vi "InitializeAOTFOutput.vi"(0 "% puls-duration":dbl=95.0, 1 "Timing Info":T2 {"#s" format="%.2e"; "Fs" format="%.2e"}, 2 "AOTF":u16(ring) items=["None", "Laser 1", "Laser 2", "Laser 1 + 2", "Laser 3", "Laser 1 + 3", "Laser 2 + 3", "Laser 1+2+3", "Laser 1+2+3+4", "Laser 2+3+4"], 3 "Image Settings":T3={"Start Position (µm)"={"x"=0.0, "y"=0.0, "z"=0.0}, "End Position (µm)"={"x"=10.0, "y"=10.0, "z"=0.0}, "Image Resolution (nm/pixel)"={"x"=50.0, "y"=50.0, "z"=100.0}, "Image Size (µm)"={"x"=10.0, "y"=10.0, "z"=0.0}, "Image Size (pixel)"={"x"=50, "y"=50, "z"=0}, "Time Resolution\n(ms/pixel)"=7.0, "1st Axis"=0, "2nd Axis"=1, "Retrace"=FALSE, "Estimated Time"=""} {"2nd Axis" items=["x", "y", "z"]; "1st Axis" items=["x", "y", "z"]; "Time Resolution\n(ms/pixel)" format="%.2f"; "Image Resolution (nm/pixel)"."z" format="%.2f"; "Image Resolution (nm/pixel)"."y" format="%.2f"; "Image Resolution (nm/pixel)"."x" format="%.2f"; "Image Size (µm)"."z" format="%.2f"; "Image Size (µm)"."y" format="%.2f"; "Image Size (µm)"."x" format="%.2f"; "End Position (µm)"."z" format="%.2f"; "End Position (µm)"."y" format="%.2f"; "End Position (µm)"."x" format="%.2f"; "Start Position (µm)"."z" format="%.2f"; "Start Position (µm)"."y" format="%.2f"; "Start Position (µm)"."x" format="%.2f"}, 4 "% rel. duration":u8=50 min=1 max=99) -> (5 "Array":T1[](array[typedef]))   [LabVIEW 2009]
uses:
  ImageSettings.ctt
  TimingInfo.ctt
  AnalogTrace.ctt
panel:
  in  "Trace":T1
  out "Frequency":dbl format="%.2e"
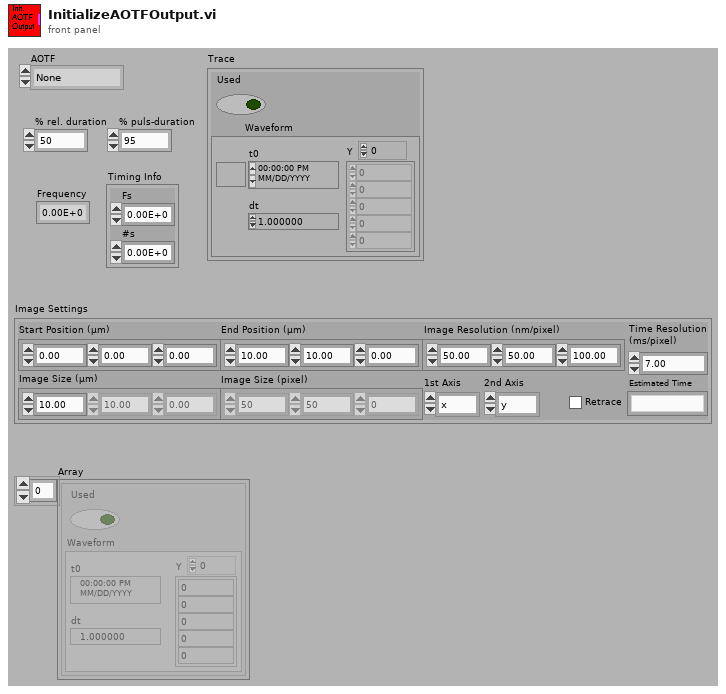
[diagram p1: front panel]
types:
  T1 = typedef "AnalogTrace.ctt" = cluster{"Used":bool, "Waveform":waveform(dbl)}
  T2 = typedef "TimingInfo.ctt" = cluster{"Fs":dbl, "#s":dbl}
  T3 = typedef "ImageSettings.ctt" = cluster{"Start Position (µm)":cluster{"x":dbl, "y":dbl, "z":dbl}, "End Position (µm)":cluster{"x":dbl, "y":dbl, "z":dbl}, "Image Resolution (nm/pixel)":cluster{"x":dbl, "y":dbl, "z":dbl}, "Image Size (µm)":cluster{"x":dbl, "y":dbl, "z":dbl}, "Image Size (pixel)":cluster{"x":u32, "y":u32, "z":u32}, "Time Resolution\n(ms/pixel)":dbl, "1st Axis":u16, "2nd Axis":u16, "Retrace":bool, "Estimated Time":string}
  T4 = typedef "AOTFSettings.ctt" = cluster{"Laser 1 Output Channel":tag, "AOTF  1 Output Voltage":dbl, "Laser 2 Output Channel":tag, "AOTF  2 Output Voltage":dbl, "Laser 3 Output Channel":tag, "AOTF  3 Output Voltage":dbl, "Pixel per Cycle":u16, "Time per Cycle  / ms":dbl, "Laser 4 Output Channel":tag, "AOTF  4 Output Voltage":dbl}
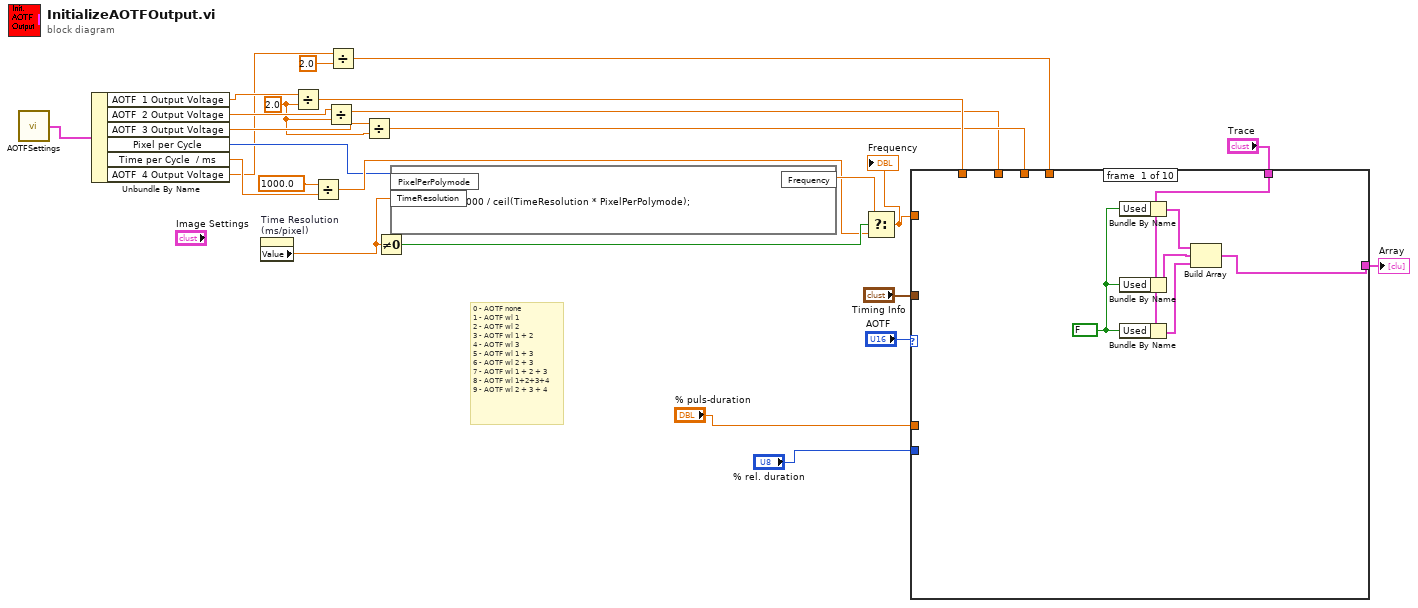
[diagram p0: block diagram]
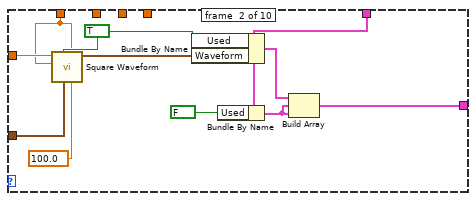
[diagram p2: hidden frame]
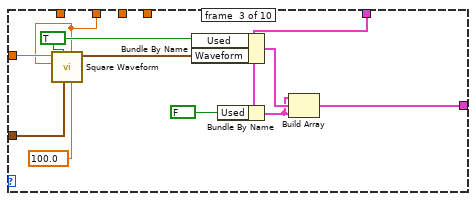
[diagram p3: hidden frame]
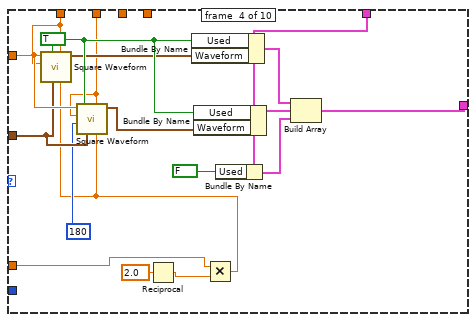
[diagram p4: hidden frame]
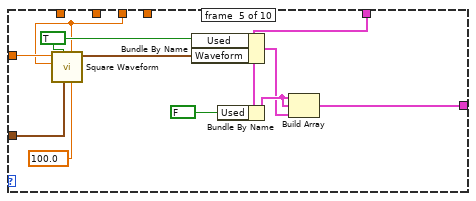
[diagram p5: hidden frame]
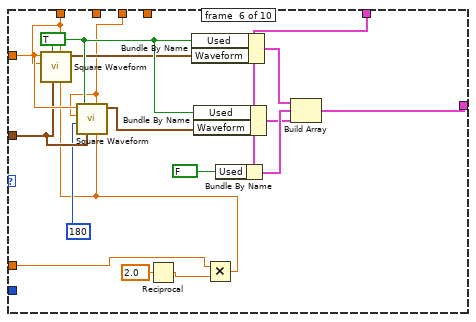
[diagram p6: hidden frame]
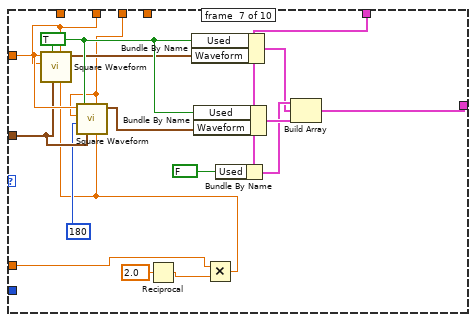
[diagram p7: hidden frame]
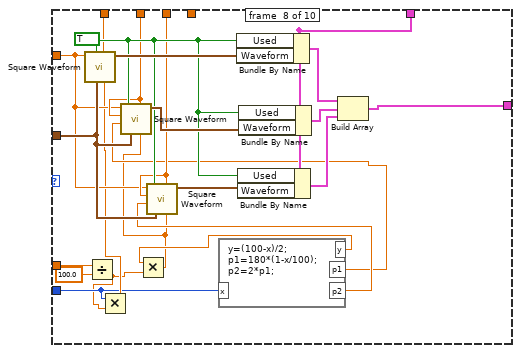
[diagram p8: hidden frame]
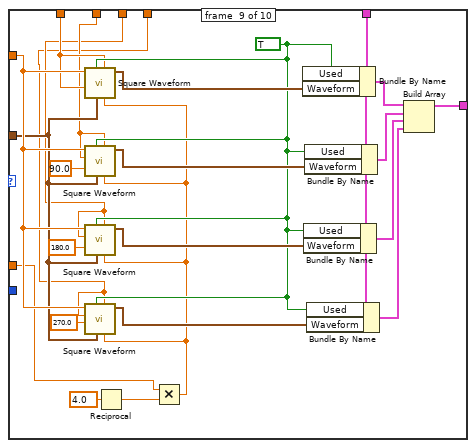
[diagram p9: hidden frame]
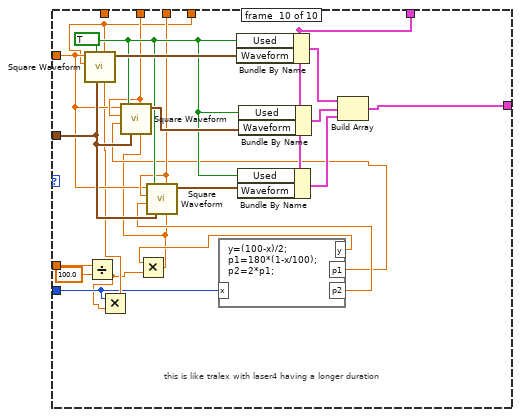
[diagram p10: hidden frame]
diagram:
  w8 = 2.0 ("y")
  # "0 - AOTF none\n1 - AOTF wl 1\n2 - AOTF wl 2\n3 - AOTF wl 1 + 2\n4 - AOTF wl 3\n5 - AOTF wl 1 + 3\n6 - AOTF wl 2 + 3\n7 - AOTF wl 1 + 2 + 3\n8 - AOTF wl 1+2+3+4\n9 - AOTF wl 2 + 3 + 4"
  n1 = call "AOTFSettings.vi"() -> ("AOTF Setting (Output)"=w16:T4)  [unwired: 2 in]
  n2 = Unbundle By Name(w16) -> ("AOTF  1 Output Voltage"=w15:dbl, "AOTF  2 Output Voltage"=w10:dbl, "AOTF  3 Output Voltage"=w12:dbl, "Pixel per Cycle"=w14:u16, "Time per Cycle  / ms"=w7:dbl, "AOTF  4 Output Voltage"=w2:dbl)
  n3 = property on="Time Resolution\n(ms/pixel)" class="Digital (strict)"() -> ("Value"=w23:dbl)  [unwired: 2 in, 2 out]
  n4 = Divide(x=w15, y=w8) -> (x/y=w13:dbl)
  n5 = Divide(x=1000.0 ("y"), y=w7) -> (x/y=w19:dbl)
  n6 = Divide(x=w10, y=w8) -> (x/y=w9:dbl)
  n7 = Divide(x=w2, y=2.0) -> (x/y=w1:dbl)
  n8 = Divide(x=w12, y=w8) -> (x/y=w11:dbl)
  n9 = Not Equal To 0?(x=w23) -> (x != 0?=w24:bool)
  n10 = formula code="Frequency =1000 / ceil(TimeResolution * PixelPerPolymode);"("PixelPerPolymode"=w14, "TimeResolution"=w23) -> ("Frequency"=w22:dbl)
  n11 = Select(t=w22, s=w24, f=w19) -> (s? t:f=w21:dbl)
  "Frequency" <- w21
  n12 = case shown="9" "AOTF" {
    tunnel: w21 -> [_ w42 w53 w71 w82 w100 w118 w130 w159 w178]
    tunnel: "Timing Info" -> [_ w41 w52 w70 w81 w99 w117 w139 w153 w186]
    tunnel: "Trace" -> [w31 w35 w47 w67 w76 w96 w114 w140 w161 w187]
    tunnel: w13 -> [_ w34 _ w62 _ w91 _ w133 w148 _]
    tunnel: [w29 w36 w48 w64 w77 w93 w112 w135 w162 w182] -> w17
    tunnel: w9 -> [_ _ w43 w61 _ _ w101 w132 w147 w180]
    tunnel: w11 -> [_ _ _ _ w72 w83 w102 w131 w146 w179]
    tunnel: "% rel. duration" -> [_ _ _ _ _ _ _ w122 _ w170]
    tunnel: "% puls-duration" -> [_ _ _ w55 _ w87 w107 w124 w150 w172]
    tunnel: w1 -> [_ _ _ _ _ _ _ _ w145 w166]
    frame #0 {
      w26 = FALSE ("Used")
      n13 = Bundle By Name(cluster=w31, "Used"=w26) -> (w30:T1)
      n14 = Bundle By Name(cluster=w31, "Used"=w26) -> (w28:T1)
      n15 = Bundle By Name(cluster=w31, "Used"=w26) -> (w27:T1)
      n16 = Build Array(w30, w28, w27) -> (w29:T1[])
    }
    frame #1 {
      w40 = TRUE ("reset signal")
      n17 = call "Square Waveform.vi"("duty cycle (%)"=100.0, "offset"=w34, "sampling info"=w41, "reset signal"=w40, "amplitude"=w34, "frequency"=w42) -> ("signal out"=w33:waveform(dbl))  [unwired: 4 in, 1 out]
      n18 = Bundle By Name(cluster=w35, "Used"=w40, "Waveform"=w33) -> (w37:T1)
      n19 = Bundle By Name(cluster=w35, "Used"=FALSE) -> (w32:T1)
      n20 = Build Array(w37, w32, w32) -> (w36:T1[])
    }
    frame #2 {
      w51 = TRUE ("reset signal")
      n21 = call "Square Waveform.vi"("duty cycle (%)"=100.0, "offset"=w43, "sampling info"=w52, "reset signal"=w51, "amplitude"=w43, "frequency"=w53) -> ("signal out"=w46:waveform(dbl))  [unwired: 4 in, 1 out]
      n22 = Bundle By Name(cluster=w47, "Used"=w51, "Waveform"=w46) -> (w45:T1)
      n23 = Bundle By Name(cluster=w47, "Used"=FALSE) -> (w44:T1)
      n24 = Build Array(w44, w45, w44) -> (w48:T1[])
    }
    frame #3 {
      w69 = TRUE ("reset signal")
      n25 = Reciprocal(x=2.0) -> (1/x=w57:dbl)
      n26 = Multiply(x=w55, y=w57) -> (x*y=w54:dbl)
      n27 = call "Square Waveform.vi"("duty cycle (%)"=w54, "offset"=w62, "sampling info"=w70, "reset signal"=w69, "amplitude"=w62, "frequency"=w71) -> ("signal out"=w68:waveform(dbl))  [unwired: 4 in, 1 out]
      n28 = call "Square Waveform.vi"("duty cycle (%)"=w54, "offset"=w61, "sampling info"=w70, "reset signal"=w69, "phase"=u8 180, "amplitude"=w61, "frequency"=w71) -> ("signal out"=w63:waveform(dbl))  [unwired: 3 in, 1 out]
      n29 = Bundle By Name(cluster=w67, "Used"=w69, "Waveform"=w68) -> (w65:T1)
      n30 = Bundle By Name(cluster=w67, "Used"=w69, "Waveform"=w63) -> (w60:T1)
      n31 = Bundle By Name(cluster=w67, "Used"=FALSE) -> (w59:T1)
      n32 = Build Array(w65, w60, w59) -> (w64:T1[])
    }
    frame #4 {
      w80 = TRUE ("reset signal")
      n33 = call "Square Waveform.vi"("duty cycle (%)"=100.0, "offset"=w72, "sampling info"=w81, "reset signal"=w80, "amplitude"=w72, "frequency"=w82) -> ("signal out"=w75:waveform(dbl))  [unwired: 4 in, 1 out]
      n34 = Bundle By Name(cluster=w76, "Used"=w80, "Waveform"=w75) -> (w73:T1)
      n35 = Bundle By Name(cluster=w76, "Used"=FALSE) -> (w74:T1)
      n36 = Build Array(w74, w74, w73) -> (w77:T1[])
    }
    frame #5 {
      w98 = TRUE ("reset signal")
      n37 = Reciprocal(x=2.0) -> (1/x=w89:dbl)
      n38 = Multiply(x=w87, y=w89) -> (x*y=w86:dbl)
      n39 = call "Square Waveform.vi"("duty cycle (%)"=w86, "offset"=w91, "sampling info"=w99, "reset signal"=w98, "amplitude"=w91, "frequency"=w100) -> ("signal out"=w97:waveform(dbl))  [unwired: 4 in, 1 out]
      n40 = call "Square Waveform.vi"("duty cycle (%)"=w86, "offset"=w83, "sampling info"=w99, "reset signal"=w98, "phase"=u8 180, "amplitude"=w83, "frequency"=w100) -> ("signal out"=w92:waveform(dbl))  [unwired: 3 in, 1 out]
      n41 = Bundle By Name(cluster=w96, "Used"=w98, "Waveform"=w97) -> (w94:T1)
      n42 = Bundle By Name(cluster=w96, "Used"=w98, "Waveform"=w92) -> (w84:T1)
      n43 = Bundle By Name(cluster=w96, "Used"=FALSE) -> (w85:T1)
      n44 = Build Array(w94, w85, w84) -> (w93:T1[])
    }
    frame #6 {
      w116 = TRUE ("reset signal")
      n45 = Reciprocal(x=2.0) -> (1/x=w109:dbl)
      n46 = Multiply(x=w107, y=w109) -> (x*y=w106:dbl)
      n47 = call "Square Waveform.vi"("duty cycle (%)"=w106, "offset"=w101, "sampling info"=w117, "reset signal"=w116, "amplitude"=w101, "frequency"=w118) -> ("signal out"=w115:waveform(dbl))  [unwired: 4 in, 1 out]
      n48 = call "Square Waveform.vi"("duty cycle (%)"=w106, "offset"=w102, "sampling info"=w117, "reset signal"=w116, "phase"=u8 180, "amplitude"=w102, "frequency"=w118) -> ("signal out"=w111:waveform(dbl))  [unwired: 3 in, 1 out]
      n49 = Bundle By Name(cluster=w114, "Used"=w116, "Waveform"=w115) -> (w103:T1)
      n50 = Bundle By Name(cluster=w114, "Used"=w116, "Waveform"=w111) -> (w105:T1)
      n51 = Bundle By Name(cluster=w114, "Used"=FALSE) -> (w104:T1)
      n52 = Build Array(w104, w103, w105) -> (w112:T1[])
    }
    frame #7 {
      w137 = TRUE ("reset signal")
      n53 = Divide(x=w124, y=100.0) -> (x/y=w121:dbl)
      n54 = Multiply(x=w122, y=w121) -> (x*y=w125:dbl)
      n55 = call "Square Waveform.vi"("duty cycle (%)"=w125, "offset"=w133, "sampling info"=w139, "reset signal"=w137, "amplitude"=w133, "frequency"=w130) -> ("signal out"=w141:waveform(dbl))  [unwired: 4 in, 1 out]
      n56 = formula code="y=(100-x)/2;\np1=180*(1-x/100);\np2=2*p1;"("x"=w122) -> ("y"=w120:dbl, "p1"=w126:dbl, "p2"=w127:dbl)
      n57 = Multiply(x=w120, y=w121) -> (x*y=w119:dbl)
      n58 = call "Square Waveform.vi"("duty cycle (%)"=w119, "offset"=w132, "sampling info"=w139, "reset signal"=w137, "phase"=w126, "amplitude"=w132, "frequency"=w130) -> ("signal out"=w138:waveform(dbl))  [unwired: 3 in, 1 out]
      n59 = call "Square Waveform.vi"("duty cycle (%)"=w119, "offset"=w131, "sampling info"=w139, "reset signal"=w137, "phase"=w127, "amplitude"=w131, "frequency"=w130) -> ("signal out"=w134:waveform(dbl))  [unwired: 3 in, 1 out]
      n60 = Bundle By Name(cluster=w140, "Used"=w137, "Waveform"=w141) -> (w136:T1)
      n61 = Bundle By Name(cluster=w140, "Used"=w137, "Waveform"=w134) -> (w129:T1)
      n62 = Bundle By Name(cluster=w140, "Used"=w137, "Waveform"=w138) -> (w128:T1)
      n63 = Build Array(w136, w128, w129) -> (w135:T1[])
    }
    frame #8 {
      w154 = TRUE
      n64 = Reciprocal(x=4.0) -> (1/x=w152:dbl)
      n65 = Multiply(x=w150, y=w152) -> (x*y=w149:dbl)
      n66 = call "Square Waveform.vi"("duty cycle (%)"=w149, "offset"=w148, "sampling info"=w153, "reset signal"=w154, "phase"=w148, "frequency"=w159) -> ("signal out"=w158:waveform(dbl))  [unwired: 4 in, 1 out]
      n67 = call "Square Waveform.vi"("duty cycle (%)"=w149, "offset"=w147, "sampling info"=w153, "reset signal"=w154, "phase"=90.0 ("amplitude"), "amplitude"=w147, "frequency"=w159) -> ("signal out"=w157:waveform(dbl))  [unwired: 3 in, 1 out]
      n68 = call "Square Waveform.vi"("duty cycle (%)"=w149, "offset"=w146, "sampling info"=w153, "reset signal"=w154, "phase"=180.0 ("amplitude"), "amplitude"=w146, "frequency"=w159) -> ("signal out"=w156:waveform(dbl))  [unwired: 3 in, 1 out]
      n69 = call "Square Waveform.vi"("duty cycle (%)"=w149, "offset"=w145, "sampling info"=w153, "reset signal"=w154, "phase"=270.0 ("amplitude"), "amplitude"=w145, "frequency"=w159) -> ("signal out"=w155:waveform(dbl))  [unwired: 3 in, 1 out]
      n70 = Bundle By Name(cluster=w161, "Used"=w154, "Waveform"=w158) -> (w163:T1)
      n71 = Bundle By Name(cluster=w161, "Used"=w154, "Waveform"=w156) -> (w164:T1)
      n72 = Bundle By Name(cluster=w161, "Used"=w154, "Waveform"=w157) -> (w165:T1)
      n73 = Bundle By Name(cluster=w161, "Used"=w154, "Waveform"=w155) -> (w160:T1)
      n74 = Build Array(w163, w165, w164, w160) -> (w162:T1[])
    }
    frame #9 {
      w184 = TRUE ("reset signal")
      # "this is like tralex with laser4 having a longer duration"
      n75 = Divide(x=w172, y=100.0) -> (x/y=w169:dbl)
      n76 = Multiply(x=w170, y=w169) -> (x*y=w173:dbl)
      n77 = call "Square Waveform.vi"("duty cycle (%)"=w173, "offset"=w166, "sampling info"=w186, "reset signal"=w184, "amplitude"=w166, "frequency"=w178) -> ("signal out"=w188:waveform(dbl))  [unwired: 4 in, 1 out]
      n78 = formula code="y=(100-x)/2;\np1=180*(1-x/100);\np2=2*p1;"("x"=w170) -> ("y"=w168:dbl, "p1"=w174:dbl, "p2"=w175:dbl)
      n79 = Multiply(x=w168, y=w169) -> (x*y=w167:dbl)
      n80 = call "Square Waveform.vi"("duty cycle (%)"=w167, "offset"=w180, "sampling info"=w186, "reset signal"=w184, "phase"=w174, "amplitude"=w180, "frequency"=w178) -> ("signal out"=w185:waveform(dbl))  [unwired: 3 in, 1 out]
      n81 = call "Square Waveform.vi"("duty cycle (%)"=w167, "offset"=w179, "sampling info"=w186, "reset signal"=w184, "phase"=w175, "amplitude"=w179, "frequency"=w178) -> ("signal out"=w181:waveform(dbl))  [unwired: 3 in, 1 out]
      n82 = Bundle By Name(cluster=w187, "Used"=w184, "Waveform"=w188) -> (w183:T1)
      n83 = Bundle By Name(cluster=w187, "Used"=w184, "Waveform"=w181) -> (w177:T1)
      n84 = Bundle By Name(cluster=w187, "Used"=w184, "Waveform"=w185) -> (w176:T1)
      n85 = Build Array(w183, w176, w177) -> (w182:T1[])
    }
  }
  "Array" <- w17
